vi "sub_sequence_enum-arr.vi"() -> (3 "HWseq-array":T1[](array[typedef]))   [LabVIEW 2019]
uses:
  Capacitor/rc-seq_enum.ctl
  _ctrl/rw.ctl
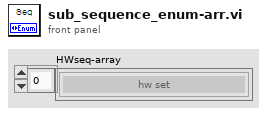
[diagram p1: front panel]
types:
  T1 = typedef "rc-seq_enum.ctl" = enum16{"hw set", "Pwr-in on", "ch-relay on", "Pwr-out on", "AO on", "AO 0v", "Pwr-in off", "Relay-all off", "Pwr-out off", "Discharge", "950 read"}
  T2 = typedef "rw.ctl" = enum16{"read", "write"}
  T3 = typedef "Testing-info.ctl" = cluster{"전체채널수":u8, "현재채널번호":u8, "Irms":dbl, "입력전압":dbl, "입력전류":dbl, "출력전압":dbl, "출력전류":dbl, "온도":dbl, "제어단 단선":bool, "제어단 단락":bool, "제어단 특성변화":bool, "출력단 단선":bool, "출력단 단락":bool, "출력단 특성변화":bool, "출력단 전압":bool, "카운트 일치":bool, "Irms 판정":bool, "온도":bool, "테스트 회수":u32, "TestType":T4, "현재회수":u32, "Ch selection":cluster{"1ch":bool, "2ch":bool, "3ch":bool, "4ch":bool, "5ch":bool, "6ch":bool}}
  T4 = typedef "sequence_single.ctl" = cluster{"Type":T5}
  T5 = typedef "Sinple-sequence-type.ctl" = enum16{"Register", "RC", "B1", "B2", "B3"}
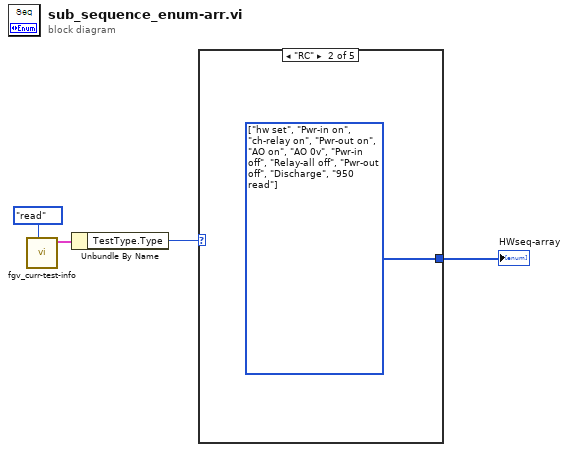
[diagram p0: block diagram]
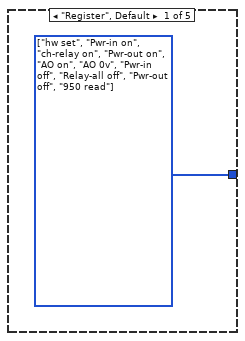
[diagram p2: hidden frame]
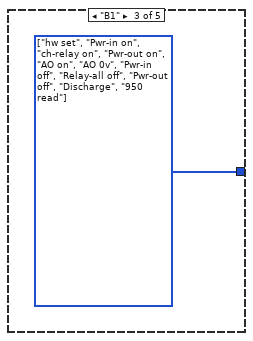
[diagram p3: hidden frame]
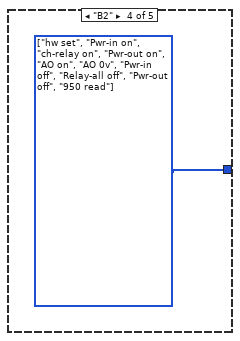
[diagram p4: hidden frame]
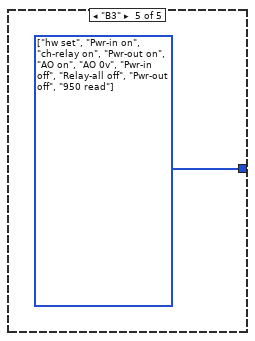
[diagram p5: hidden frame]
diagram:
  n1 = call "fgv_curr-test-info.vi"("cmd"=rw."read") -> ("현재테스트 정보 2"=w2:T3)  [unwired: 10 in]
  n2 = Unbundle By Name(w2) -> ("TestType.Type"=w1:T5)
  n3 = case shown="\"RC\"" w1 {
    tunnel: [w5 w6 w7 w8 w9] -> w4
    frame "Register", Default {
      w5 = T1[] [enum."hw set", enum."Pwr-in on", enum."ch-relay on", enum."Pwr-out on", enum."AO on", enum."AO 0v", enum."Pwr-in off", enum."Relay-all off", enum."Pwr-out off", enum."950 read"] items=["hw set", "Pwr-in on", "ch-relay on", "Pwr-out on", "AO on", "AO 0v", "Pwr-in off", "Relay-all off", "Pwr-out off", "Discharge", "950 read"]
    }
    frame "RC" {
      w6 = T1[] [enum."hw set", enum."Pwr-in on", enum."ch-relay on", enum."Pwr-out on", enum."AO on", enum."AO 0v", enum."Pwr-in off", enum."Relay-all off", enum."Pwr-out off", enum."Discharge", enum."950 read"] items=["hw set", "Pwr-in on", "ch-relay on", "Pwr-out on", "AO on", "AO 0v", "Pwr-in off", "Relay-all off", "Pwr-out off", "Discharge", "950 read"]
    }
    frame "B1" {
      w7 = T1[] [enum."hw set", enum."Pwr-in on", enum."ch-relay on", enum."Pwr-out on", enum."AO on", enum."AO 0v", enum."Pwr-in off", enum."Relay-all off", enum."Pwr-out off", enum."Discharge", enum."950 read"] items=["hw set", "Pwr-in on", "ch-relay on", "Pwr-out on", "AO on", "AO 0v", "Pwr-in off", "Relay-all off", "Pwr-out off", "Discharge", "950 read"]
    }
    frame "B2" {
      w8 = T1[] [enum."hw set", enum."Pwr-in on", enum."ch-relay on", enum."Pwr-out on", enum."AO on", enum."AO 0v", enum."Pwr-in off", enum."Relay-all off", enum."Pwr-out off", enum."950 read"] items=["hw set", "Pwr-in on", "ch-relay on", "Pwr-out on", "AO on", "AO 0v", "Pwr-in off", "Relay-all off", "Pwr-out off", "Discharge", "950 read"]
    }
    frame "B3" {
      w9 = T1[] [enum."hw set", enum."Pwr-in on", enum."ch-relay on", enum."Pwr-out on", enum."AO on", enum."AO 0v", enum."Pwr-in off", enum."Relay-all off", enum."Pwr-out off", enum."950 read"] items=["hw set", "Pwr-in on", "ch-relay on", "Pwr-out on", "AO on", "AO 0v", "Pwr-in off", "Relay-all off", "Pwr-out off", "Discharge", "950 read"]
    }
  }
  "HWseq-array" <- w4
